vi "TriggeredFrequencySweep3.vi"() -> ()   [LabVIEW 2020]
uses:
  <vilib>/DAQmx/read.llb/DAQmx Read (Digital Bool 1Line 1Point).vi
  <vilib>/DAQmx/read.llb/DAQmx Read (Analog 1D Wfm NChan NSamp).vi
  <vilib>/DAQmx/create/channels.llb/DAQmx Create Channel (AI-Acceleration-Accelerometer).vi
  <vilib>/DAQmx/configure/timing.llb/DAQmx Timing (Sample Clock).vi
  <vilib>/DAQmx/miscellaneous.llb/DAQmx Fill In Error Info.vi
  <vilib>/express/express analysis/Spectral/Block/exnSpectralBlock spectral measurements RMS poly.vi
  <vilib>/express/express analysis/Spectral/Block/exnSpectralBlock spectral measurements RMS array WFM.vi
  <vilib>/express/express analysis/Spectral/XNode/ExpressSpectralMeasurementsBlockNode.xnode
  <resource>/objmgr/daqmx.rc
panel:
  in  "stop 3":bool caption="stop"
  out "data 4":waveform(dbl)[](graph) caption="data"
  out "data 2":cluster{"f0":dbl, "df":dbl, "magnitude":dbl[]}[](graph) caption="data"
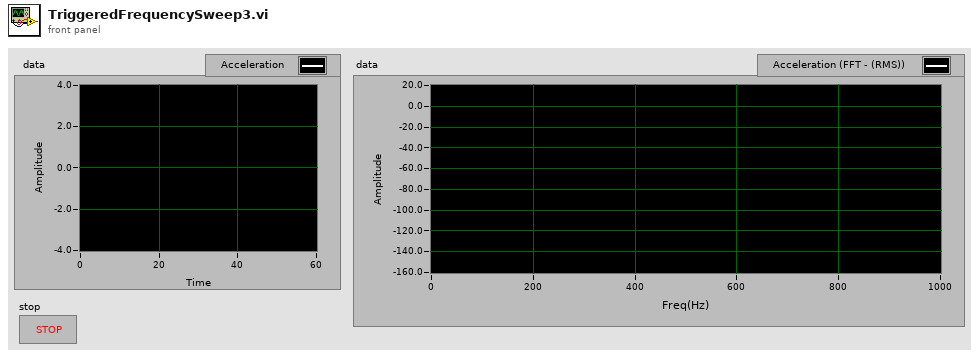
[diagram p1: front panel]
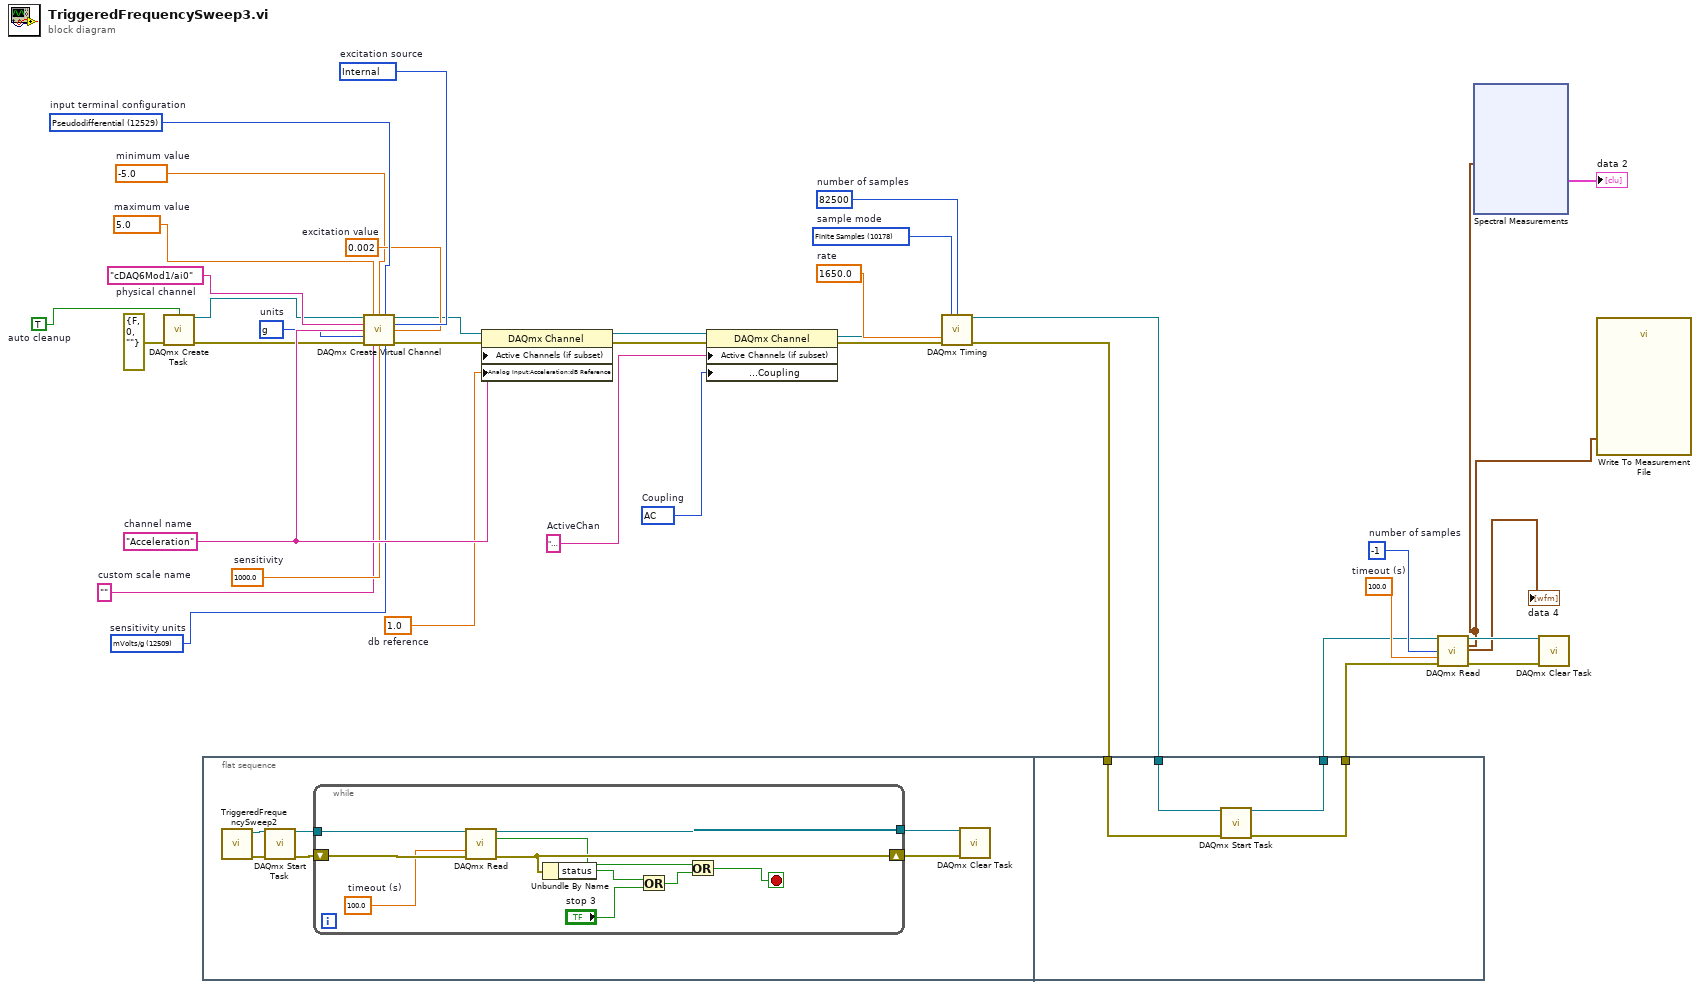
[diagram p0: block diagram]
diagram:
  w31 = 10178 items=["Finite Samples"=10178, "Continuous Samples"=10123, "Hardware Timed Single Point"=12522]  # sample mode
  w30 = 82500  # number of samples
  w29 = 1650.0  # rate
  w25 = 10045 items=["AC"=10045, "DC"=10050, "GND"=10066]  # Coupling
  w24 = "Acceleration"  # ActiveChan
  w22 = 1.0  # db reference
  w19 = 10186 items=["g"=10186, "m/s^2"=12470, "From Custom Scale"=10065]  # units
  w18 = 12529 items=["default"=-1, "RSE"=10083, "NRSE"=10078, "Differential"=10106, "Pseudodifferential"=12529]  # input terminal configuration
  w17 = 10200 items=["Internal"=10200, "External"=10167, "None"=10230]  # excitation source
  w16 = 0.002  # excitation value
  w15 = 12509 items=["mVolts/g"=12509, "Volts/g"=12510]  # sensitivity units
  w14 = 1000.0  # sensitivity
  w23 = "Acceleration"  # channel name
  w12 = ""  # custom scale name
  w11 = -5.0  # minimum value
  w10 = 5.0  # maximum value
  w9 = "cDAQ6Mod1/ai0"  # physical channel
  w7 = TRUE  # auto cleanup
  w35 = 100.0  # timeout (s)
  w36 = -1  # number of samples
  n1 = call <vilib>:"DAQmx Create Task.vi"("auto cleanup"=w7, "error in"=errorcluster {"status"=FALSE, "code"=0, "source"=""}) -> ("task out"=w8:refnum<k21>, "error out"=w6:errorcluster)  [unwired: 12 in]
  n2 = flat-sequence {
    tunnel: w5 -> [w57]
    tunnel: w4 -> [w56]
    tunnel: [w55] -> w3
    tunnel: [w54] -> w2
    frame #0 {
      n3 = call "TriggeredFrequencySweep2.vi"() -> ("error out"=w38:errorcluster, "task out"=w39:refnum<k21>)  [unwired: 10 in]
      n4 = call <vilib>:"DAQmx Start Task.vi"("task/channels in"=w39, "error in"=w38) -> ("task out"=w43:refnum<k21>, "error out"=w42:errorcluster)  [unwired: 12 in]
      n5 = while {
        tunnel: w43 -> [w53]
        tunnel: [w51] -> w40
        shift-right: [w49] -> w41
        shift-left: w42 -> [w52]
        stop <- w46 stop-if-true
        w47 = 100.0  # timeout (s)
        n6 = call-poly <vilib>:"DAQmx Read.vi"("task/channels in"=w53, "timeout"=w47, "error in"=w52) -> ("task out"=w51:refnum<k21>, "data"=w44:bool, "error out"=w49:errorcluster)  [unwired: 10 in]
        n7 = Unbundle By Name(w49) -> ("status"=w50:bool)
        n8 = Or(x=w50, y="stop 3") -> (x .or. y?=w45:bool)
        n9 = Or(x=w44, y=w45) -> (x .or. y?=w46:bool)
      }
      n10 = call <vilib>:"DAQmx Clear Task.vi"("task in"=w40, "error in"=w41) -> ()  [unwired: 13 in, 1 out]
    }
    frame #1 {
      n11 = call <vilib>:"DAQmx Start Task.vi"("task/channels in"=w57, "error in"=w56) -> ("task out"=w55:refnum<k21>, "error out"=w54:errorcluster)  [unwired: 12 in]
    }
  }
  n12 = call-poly <vilib>:"DAQmx Create Virtual Channel.vi"("task in"=w8, "maximum value"=w10, "minimum value"=w11, "input terminal configuration"=w18, "physical channels"=w9, "current excitation source"=w17, "name to assign"=w23, "current excitation value"=w16, "units"=w19, "error in"=w6, "custom scale name"=w12, "sensitivity"=w14, "sensitivity units"=w15) -> ("task out"=w13:refnum<k21>, "error out"=w20:errorcluster)  [unwired: 1 in]
  n13 = property class="DAQmx Channel"(reference=w13, error in=w20, "Active Channels (if subset)"=w23, "Analog Input:Acceleration:dB Reference"=w22) -> (reference out=w27:refnum<k21>, error out=w21:errorcluster)
  n14 = property class="DAQmx Channel"(reference=w27, error in=w21, "Active Channels (if subset)"=w24, "Analog Input:General Properties:Input Configuration:Coupling"=w25) -> (reference out=w28:refnum<k21>, error out=w26:errorcluster)
  n15 = call-poly <vilib>:"DAQmx Timing.vi"("task/channels in"=w28, "sample mode"=w31, "samples per channel"=w30, "rate"=w29, "error in"=w26) -> ("task out"=w5:refnum<k21>, "error out"=w4:errorcluster)  [unwired: 9 in]
  n16 = call-poly <vilib>:"DAQmx Read.vi"("task/channels in"=w3, "number of samples per channel"=w36, "timeout"=w35, "error in"=w2) -> ("task out"=w33:refnum<k21>, "data"=w1:waveform(dbl)[], "error out"=w34:errorcluster)  [unwired: 9 in]
  "data 4" <- w1
  n17 = xnode "Spectral Measurements"("Signals"=w1) -> ("FFT - (RMS)"=→"data 2":cluster{"f0":dbl, "df":dbl, "magnitude":dbl[]}[])  [unwired: 1 in, 2 out]
  n18 = call <vilib>:"DAQmx Clear Task.vi"("task in"=w33, "error in"=w34) -> ()  [unwired: 13 in, 1 out]
  n19 = call "Write To Measurement File"("Signals"=w1) -> ()  [unwired: 16 in, 3 out]
